vi "Serial Delay(msec).vi"(8 "에러 입력(에러 없음)":errorcluster, 10 "milliseconds to wait":u32, 11 "VISA 참조 번호 입력":refnum<visa-resource-name>) -> (0 "에러 출력":errorcluster, 3 "VISA 참조 번호 출력":refnum<visa-resource-name>)   [LabVIEW 2014]
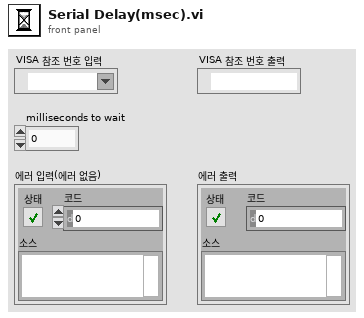
[diagram p1: front panel]
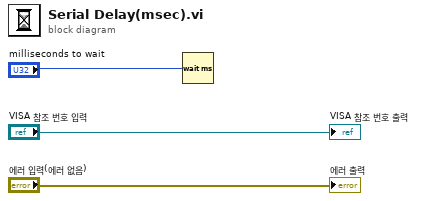
[diagram p0: block diagram]
diagram:
  n1 = Wait (ms)(milliseconds to wait="milliseconds to wait") -> ()  [unwired: 1 out]
  "VISA 참조 번호 출력" <- "VISA 참조 번호 입력"
  "에러 출력" <- "에러 입력(에러 없음)"
